vi "Update Check-out Details.vi"(0 "Guest Manager Model in":refnum<class "Guest Manager Model.lvclass">, 5 "Guest Contact Number":string, 7 "Primary Guest Name":string, 9 "Bill Summary":string, 11 "error in (no error)":errorcluster) -> (4 "Guest Manager Model out":refnum<class "Guest Manager Model.lvclass">, 15 "error out":errorcluster)   [LabVIEW 2023, in "Guest Manager Model.lvlib" / "Guest Manager Model.lvclass"]
uses:
  Guest Manager Model.lvclass
  Guest Manager Model.lvclass/Guest Manager Model.ctl
  Guest Manager UI/Guest Manager UI Messages/Update Check-out Details Msg/Update Check-out Details Msg.lvclass
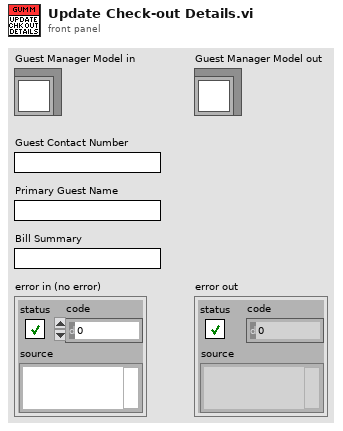
[diagram p1: front panel]
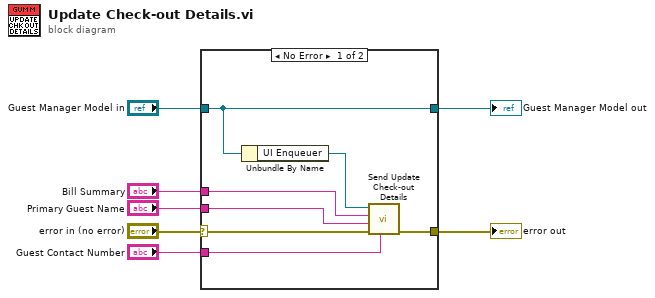
[diagram p0: block diagram]
diagram:
  n1 = case shown="No Error" "error in (no error)" {
    selector: "error in (no error)" -> [w14 w16]
    tunnel: [w13 w16] -> w6
    tunnel: [w11 w15] -> w4
    tunnel: "Guest Manager Model in" -> [w11 w15]
    tunnel: "Bill Summary" -> [w12 _]
    tunnel: "Primary Guest Name" -> [w9 _]
    tunnel: "Guest Contact Number" -> [w8 _]
    frame No Error {
      n2 = Unbundle By Name(w11) -> ("UI Enqueuer"=w10:refnum<class "Message Enqueuer.lvclass">)
      n3 = call "Send Update Check-out Details.vi"("Guest Contact Number"=w8, "error in (no error)"=w14, "Primary Guest Name"=w9, "Bill Summary"=w12, "Message Enqueuer"=w10) -> ("error out"=w13:errorcluster)  [unwired: 5 in, 1 out]
    }
    frame Error {
    }
  }
  "error out" <- w6
  "Guest Manager Model out" <- w4
